vi "move to relative xy position.vi"(10 "setY":dbl, 11 "setX":dbl) -> ()   [LabVIEW 2012]
doc: "SciScan 1.2 160622"
uses:
  GFG/GFGnumericGet.vi
  GFG/GFGbooleanGet.vi
  GFG/GFG library.lvlib
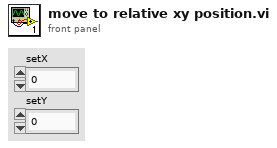
[diagram p1: front panel]
types:
  T1 = cluster{"Xoffset":dbl, "Yoffset":dbl, "Zoffset":dbl}
  T2 = cluster{"moveXabs":dbl, "moveYabs":dbl, "moveZabs":dbl}
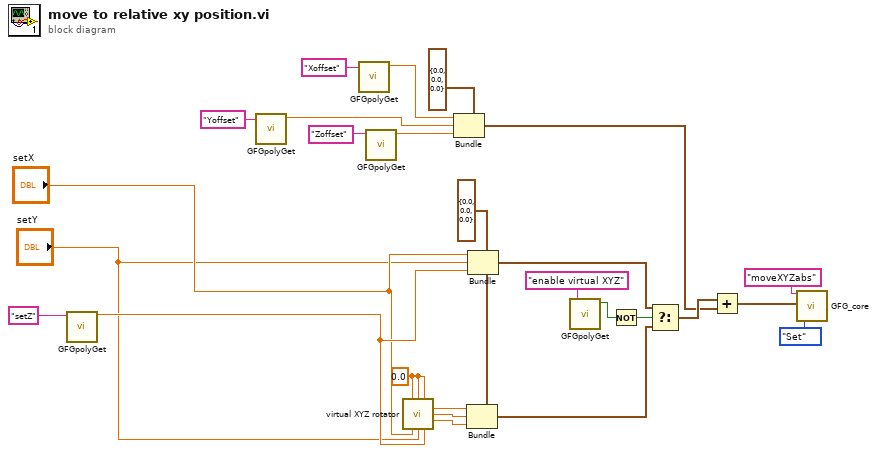
[diagram p0: block diagram]
diagram:
  w16 = 0.0 ("current pos X")
  w21 = T2 {"moveXabs"=0.0, "moveYabs"=0.0, "moveZabs"=0.0} ("output cluster")
  n1 = call-poly "GFGpolyGet.vi"("Variable Name in"="setZ") -> ("Numeric"=w12:dbl)  [unwired: 8 in, 2 out]
  n2 = call-poly "GFGpolyGet.vi"("Variable Name in"="Yoffset") -> ("Numeric"=w5:dbl)  [unwired: 8 in, 2 out]
  n3 = call-poly "GFGpolyGet.vi"("Variable Name in"="Xoffset") -> ("Numeric"=w6:dbl)  [unwired: 8 in, 2 out]
  n4 = call-poly "GFGpolyGet.vi"("Variable Name in"="Zoffset") -> ("Numeric"=w4:dbl)  [unwired: 8 in, 2 out]
  n5 = call "virtual XYZ rotator.vi"("current pos X"=w16, "current pos Y"=w16, "current pos Z"=w16, "virtual X relative"="setX", "virtual Y relative"="setY", "virtual Z relative"=w12) -> ("new pos X"=w24:dbl, "new pos Y"=w23:dbl, "new pos Z"=w22:dbl)  [unwired: 7 in]
  n6 = Bundle(cluster=T1 {"Xoffset"=0.0, "Yoffset"=0.0, "Zoffset"=0.0} ("output cluster"), "Xoffset"=w6, "Yoffset"=w5, "Zoffset"=w4) -> (w3:T1)
  n7 = Bundle(cluster=w21, "moveXabs"=w24, "moveYabs"=w23, "moveZabs"=w22) -> (w19:T2)
  n8 = Bundle(cluster=w21, "moveXabs"="setX", "moveYabs"="setY", "moveZabs"=w12) -> (w20:T2)
  n9 = call-poly "GFGpolyGet.vi"("Variable Name in"="enable virtual XYZ") -> ("Boolean Value OUT"=w18:bool)  [unwired: 9 in, 1 out]
  n10 = Not(x=w18) -> (.not. x?=w17:bool)
  n11 = Select(t=w20, s=w17, f=w19) -> (s? t:f=w13:T2)
  n12 = Add(x=w13, y=w3) -> (x+y=w11:cluster{dbl, dbl, dbl})
  n13 = call "GFG_core.vi"("Variable Name in"="moveXYZabs", "Variant in"=w11, "Action"=enum16{"Init", "Set", "Get"}."Set") -> ()  [unwired: 10 in, 7 out]
